vi "CRYCalibration Value Replace.vi"(9 "Step No.":i32, 10 "Corr/EQ/Sens Name":string, 11 "Type":enum16{"Curves", "Values", "Results", "WFM"}(ring)) -> ()   [LabVIEW 2013]
uses:
  CRYCal Global.vi
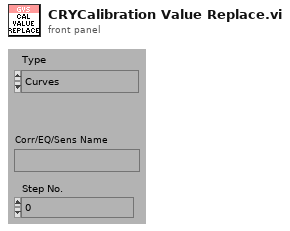
[diagram p1: front panel]
types:
  T1 = typedef "CRYData Cluster.ctl" = cluster{"Name":string, "Curve":cluster{"x":dbl, "y":dbl, "z":dbl}[], "X data":u16, "Y data":u16, "Z data":u16, "X axis":u16, "Y axis":u16, "Z axis":u16, "X unit":string, "Y unit":string, "Z unit":string, "X dB ref":dbl, "Y dB ref":dbl, "Z dB ref":dbl, "single val":bool, "protected":bool, "display X":bool, "display Y":bool, "display Z":bool, "Test Info":string, "Step No.":i32, "Plot Settings":cluster{"Color":u32, "Interpolation":u8, "Point Style":u8, "Line Style":u8, "Point Color":u32, "Line Width":u8, "Bar Plot Style":u8, "Fill To":i16}, "AutoProtect":bool}
  T2 = typedef "CRYCalibration All Cluster.ctl" = cluster{"Calibration 2D":T3[], "Help":string, "Tab Value":i32, "Input Signal Type":string, "Output Signal Type":string}
  T3 = typedef "CRYCalibration 2DCluster.ctl" = cluster{"Calibration":T4, "Corr Curve":T1, "EQ Curve":T1, "Sens Curve":T1}
  T4 = typedef "CRYCalibration Cluster.ctl" = cluster{"Calibration Step Name":string, "Device":string, "Correction Curve Name":string, "Equalization Curve Name":string, "Sensitivity Curve Name":string, "Corr Folder and File":string, "EQ Folder and File":string, "Sens Folder and File":string, "Corr Step size":u16, "EQ Step size":u16, "Input":bool, "Last Cal Date (sec)":timestamp, "Cha Name":string, "Corr Curve Found":bool, "EQ Curve Found":bool, "Sens Curve Found":bool, "Signal Type":string, "Calibrated Device":string, "Hz":u32}
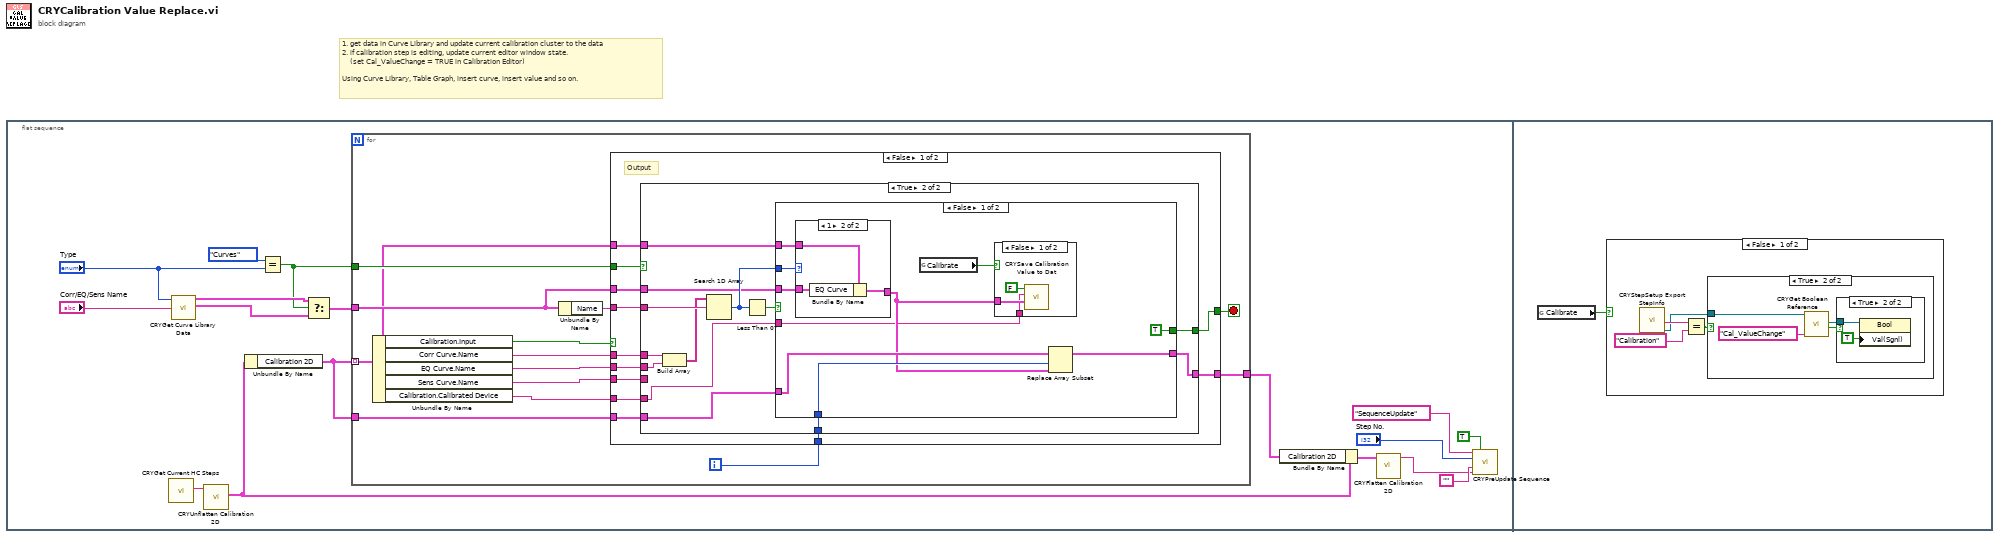
[diagram p0: block diagram]
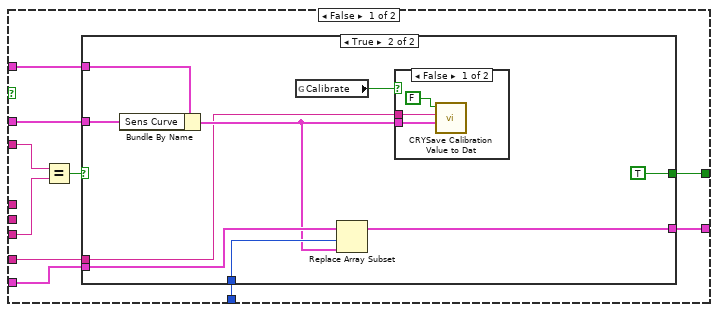
[diagram p2: hidden frame]
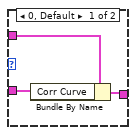
[diagram p6: hidden frame]
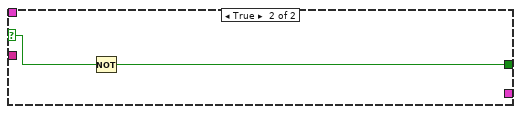
[diagram p7: hidden frame]
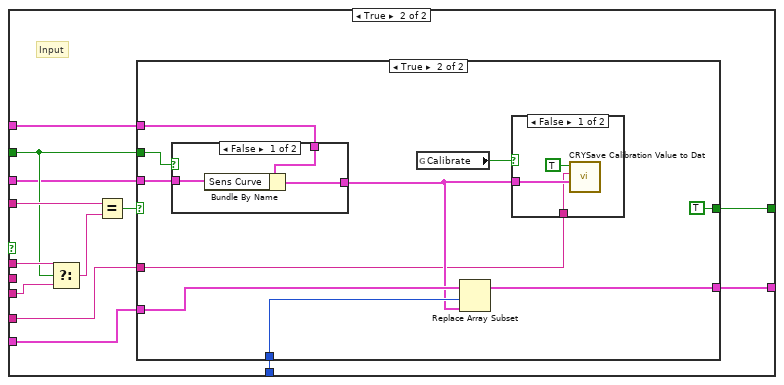
[diagram p8: hidden frame]
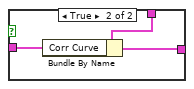
[diagram p11: hidden frame]
diagram:
  # "1. get data in Curve Library and update current calibration cluster to the data\n2. if calibration step is editing, update current editor window state.\n    (set Cal_ValueChange = TRUE in Calibration Editor)\n\nUsing Curve Library, Table Graph, insert curve, insert value and so on."
  n1 = flat-sequence {
    frame #0 {
      n2 = call "CRYGet Current HC Steps.vi"() -> ("Calibration setup flattened Out"=w3:string)  [unwired: 10 in, 1 out]
      n3 = call "CRYGet Curve Library Data.vi"("Type"="Type", "Data Name"="Corr/EQ/Sens Name") -> ("Curve"=w10:T1, "Value"=w9:T1)  [unwired: 3 out]
      n4 = call "CRYUnflatten Calibration 2D.vi"("Flattened Calibration"=w3) -> ("Calibration Step Out"=w5:T2)  [unwired: 2 in, 8 out]
      n5 = Unbundle By Name(w5) -> ("Calibration 2D"=w6:T3[])
      n6 = Equal?(x=enum16{"Curves", "Values", "Results", "WFM"}."Curves", y="Type") -> (x = y?=w8:bool)
      n7 = Select(t=w10, s=w8, f=w9) -> (s? t:f=w7:T1)
      n8 = for {
        tunnel: w6 -> [w21] mode=indexing
        tunnel: w8 -> [w26]
        tunnel: w7 -> [w23]
        tunnel: w6 -> [w22]
        tunnel: [w19] -> w1
        i -> [w20]
        stop <- w25 stop-if-true
        n9 = Unbundle By Name(w21) -> ("Calibration.Input"=w30:bool, "Corr Curve.Name"=w29:string, "EQ Curve.Name"=w28:string, "Sens Curve.Name"=w27:string, "Calibration.Calibrated Device"=w18:string)
        n10 = Unbundle By Name(w23) -> ("Name"=w24:string)
        n11 = case shown="False" w30 {
          tunnel: w29 -> [w33 w111]
          tunnel: w28 -> [w32 _]
          tunnel: w27 -> [w40 w110]
          tunnel: w26 -> [w42 w106]
          tunnel: w24 -> [w41 w112]
          tunnel: [w39 w107] -> w25
          tunnel: w23 -> [w37 w105]
          tunnel: w22 -> [w36 w104]
          tunnel: w21 -> [w38 w103]
          tunnel: w20 -> [w35 w102]
          tunnel: [w34 w101] -> w19
          tunnel: w18 -> [w31 w100]
          frame False {
            # "Output"
            n12 = case shown="True" w42 {
              tunnel: w41 -> [w52 w76]
              tunnel: w40 -> [w51 _]
              tunnel: [w49 w73] -> w39
              tunnel: w38 -> [w48 w70]
              tunnel: w37 -> [w47 w71]
              tunnel: w36 -> [w46 w69]
              tunnel: w35 -> [w45 w68]
              tunnel: [w44 w67] -> w34
              tunnel: w33 -> [_ w78]
              tunnel: w32 -> [_ w77]
              tunnel: w31 -> [w43 w66]
              frame False {
                n13 = Equal?(x=w52, y=w51) -> (x = y?=w50:bool)
                n14 = case shown="True" w50 {
                  selector: w50 -> [w53 _]
                  tunnel: [w53 TRUE] -> w49
                  tunnel: w48 -> [_ w61]
                  tunnel: w47 -> [_ w60]
                  tunnel: w46 -> [_ w59]
                  tunnel: w45 -> [_ w58]
                  tunnel: [_ w57] -> w44
                  tunnel: w43 -> [_ w55]
                  frame False {
                  }
                  frame True {
                    n15 = Bundle By Name(cluster=w61, "Sens Curve"=w60) -> (w56:T3)
                    n16 = global read "CRYCal Global.vi" "Calibrate"() -> (w54:bool)
                    n17 = Replace Array Subset(array=w59, new element=w56, index=w58) -> (w57:T3[])
                    n18 = case shown="False" w54 {
                      tunnel: w56 -> [w64 _]
                      tunnel: w55 -> [w63 _]
                      frame False {
                        n19 = call "CRYSave Calibration Value to Dat.vi"("Calibration 2D Cluster"=w64, "Calibrated Device"=w63, "Input"=FALSE) -> ()  [unwired: 9 in]
                      }
                      frame True {
                      }
                    }
                  }
                }
              }
              frame True {
                n20 = Build Array(w78, w77) -> (w75:string[])
                n21 = Search 1D Array(1D array=w75, element=w76) -> (index of element=w72:i32)  [unwired: 1 in]
                n22 = Less Than 0?(x=w72) -> (x < 0?=w74:bool)
                n23 = case shown="False" w74 {
                  selector: w74 -> [_ w99]
                  tunnel: [TRUE w98] -> w73
                  tunnel: w72 -> [w88 _]
                  tunnel: w71 -> [w87 _]
                  tunnel: w70 -> [w86 _]
                  tunnel: w69 -> [w85 _]
                  tunnel: w68 -> [w84 _]
                  tunnel: [w83 _] -> w67
                  tunnel: w66 -> [w80 _]
                  frame False {
                    n24 = case shown="1" w88 {
                      tunnel: w87 -> [w93 w96]
                      tunnel: w86 -> [w94 w97]
                      tunnel: [w92 w95] -> w81
                      frame 0, Default {
                        n25 = Bundle By Name(cluster=w94, "Corr Curve"=w93) -> (w92:T3)
                      }
                      frame 1 {
                        n26 = Bundle By Name(cluster=w97, "EQ Curve"=w96) -> (w95:T3)
                      }
                    }
                    n27 = global read "CRYCal Global.vi" "Calibrate"() -> (w79:bool)
                    n28 = case shown="False" w79 {
                      tunnel: w81 -> [w91 _]
                      tunnel: w80 -> [w90 _]
                      frame False {
                        n29 = call "CRYSave Calibration Value to Dat.vi"("Calibration 2D Cluster"=w91, "Calibrated Device"=w90, "Input"=FALSE) -> ()  [unwired: 9 in]
                      }
                      frame True {
                      }
                    }
                    n30 = Replace Array Subset(array=w85, new element=w81, index=w84) -> (w83:T3[])
                  }
                  frame True {
                    n31 = Not(x=w99) -> (.not. x?=w98:bool)
                  }
                }
              }
            }
          }
          frame True {
            # "Input"
            n32 = Select(t=w111, s=w106, f=w110) -> (s? t:f=w109:string)
            n33 = Equal?(x=w112, y=w109) -> (x = y?=w108:bool)
            n34 = case shown="True" w108 {
              selector: w108 -> [w113 _]
              tunnel: [w113 TRUE] -> w107
              tunnel: w106 -> [_ w123]
              tunnel: w105 -> [_ w121]
              tunnel: w104 -> [_ w120]
              tunnel: w103 -> [_ w122]
              tunnel: w102 -> [_ w119]
              tunnel: [_ w117] -> w101
              tunnel: w100 -> [_ w115]
              frame False {
              }
              frame True {
                n35 = case shown="False" w123 {
                  tunnel: w122 -> [w129 w132]
                  tunnel: w121 -> [w128 w131]
                  tunnel: [w127 w130] -> w116
                  frame False {
                    n36 = Bundle By Name(cluster=w129, "Sens Curve"=w128) -> (w127:T3)
                  }
                  frame True {
                    n37 = Bundle By Name(cluster=w132, "Corr Curve"=w131) -> (w130:T3)
                  }
                }
                n38 = global read "CRYCal Global.vi" "Calibrate"() -> (w114:bool)
                n39 = Replace Array Subset(array=w120, new element=w116, index=w119) -> (w117:T3[])
                n40 = case shown="False" w114 {
                  tunnel: w116 -> [w125 _]
                  tunnel: w115 -> [w124 _]
                  frame False {
                    n41 = call "CRYSave Calibration Value to Dat.vi"("Calibration 2D Cluster"=w125, "Calibrated Device"=w124, "Input"=TRUE) -> ()  [unwired: 9 in]
                  }
                  frame True {
                  }
                }
              }
            }
          }
        }
      }
      n42 = Bundle By Name(cluster=w5, "Calibration 2D"=w1) -> (w4:T2)
      n43 = call "CRYFlatten Calibration 2D.vi"("Calibration All Cluster"=w4) -> ("Calibration flattened"=w13:string)  [unwired: 10 out]
      n44 = call "CRYPreUpdate Sequence.vi"("EventName"="SequenceUpdate", "Proper VI No"="Step No.", "Project View Step Name Identifier Arg1"="", "Step flattened Arg2"=w13, "AllChangeFlg"=TRUE ("Name/Identifier")) -> ()  [unwired: 11 in]
    }
    frame #1 {
      n45 = global read "CRYCal Global.vi" "Calibrate"() -> (w133:bool)
      n46 = case shown="False" w133 {
        frame False {
          n47 = call "CRYStepSetup Export StepInfo.vi"() -> ("pVIRef"=w134:refnum<vi>, "sCategory"=w136:string)  [unwired: 9 in, 1 out]
          n48 = Equal?(x=w136, y="Calibration") -> (x = y?=w135:bool)
          n49 = case shown="True" w135 {
            tunnel: w134 -> [_ w139]
            frame False {
            }
            frame True {
              n50 = call "CRYGet Boolean Reference.vi"("Label Name"="Cal_ValueChange", "VI Refnum"=w139) -> ("Exist?"=w138:bool, "Boolean Ref"=w140:refnum<vi>)  [unwired: 7 in, 1 out]
              n51 = case shown="True" w138 {
                tunnel: w140 -> [_ w143]
                frame False {
                }
                frame True {
                  n52 = property class="Bool"(reference=w143, "Val(Sgnl)"=TRUE) -> ()  [unwired: 1 in, 2 out]
                }
              }
            }
          }
        }
        frame True {
        }
      }
    }
  }
